vi "TCP Server UnRegister Connection Handler.vi"(8 "error in (no error)":errorcluster, 10 "connection ID":refnum<k5>, 11 "TCP Server RefNum":refnum<class "JKI TCP Server.lvclass">) -> (0 "error out":errorcluster, 1 "Connection Info":T3, 2 "VI References":T2)   [LabVIEW 2020, in "JKI TCP Server.lvclass"]
uses:
  JKI TCP Server.lvclass
  _Data Structures/TCP Server Connection Info Cluster.ctl
  _Data Structures/TCP Server Handler RefNum.ctl
panel:
  # "Copyright © 2004-2008 JKI. All rights reserved.\n\nAuthor: Jim Kring [jim.kring@jameskring.com]\n\nThis library is provided \"AS IS\" ,WITHOUT WARRANTIES OR \nCONDITIONS OF ANY KIND, either express or implied.\n\nJames Kring, Inc. -- http://www.jameskring.com"
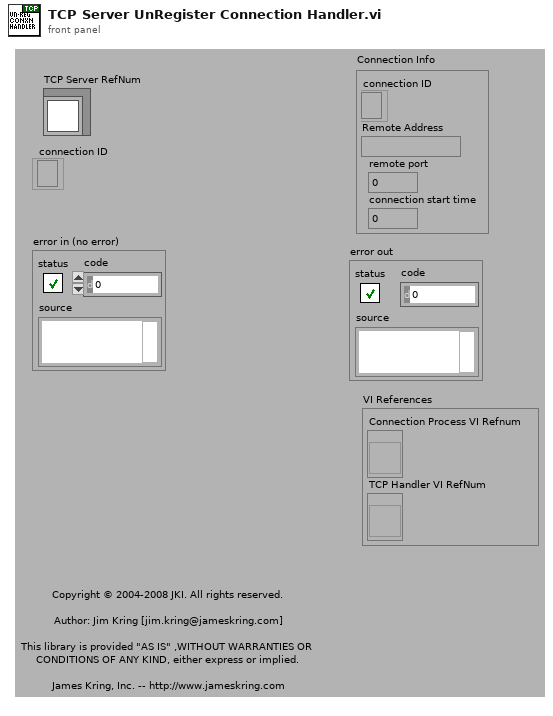
[diagram p1: front panel]
types:
  T1 = typedef "JKI TCP Server.lvclass/TCP Server Handler RefNum.ctl" = refnum<vi>
  T2 = cluster{"Connection Process VI Refnum":refnum<vi>, "TCP Handler VI RefNum":T1}
  T3 = typedef "JKI TCP Server.lvclass/TCP Server Connection Info Cluster.ctl" = cluster{"connection ID":refnum<k5>, "Remote Address":string, "remote port":u16, "connection start time":u32}
  T4 = typedef "JKI TCP Server.lvclass/TCP Server Data.ctl" = cluster{"Listener Info":T5, "Connection Process VI RefNums":refnum<vi>[], "dup connection IDs (for quick search)":refnum<k5>[], "Connections":T3[], "Connection Handler VI Path":path, "Handler Is Reentrant?":bool, "TCP Handler Instance RefNums":T1[], "TCP Handler VI RefNum":T1, "No. Connections":u32, "Max Connections":u32, "server start time":u32, "Additional Data":variant}
  T5 = typedef "JKI TCP Server.lvclass/TCP Server Listener Info Cluster.ctl" = cluster{"listener ID":refnum<k5>, "net address":u32, "port":u16, "Listener Process VI Refnum":refnum<vi>}
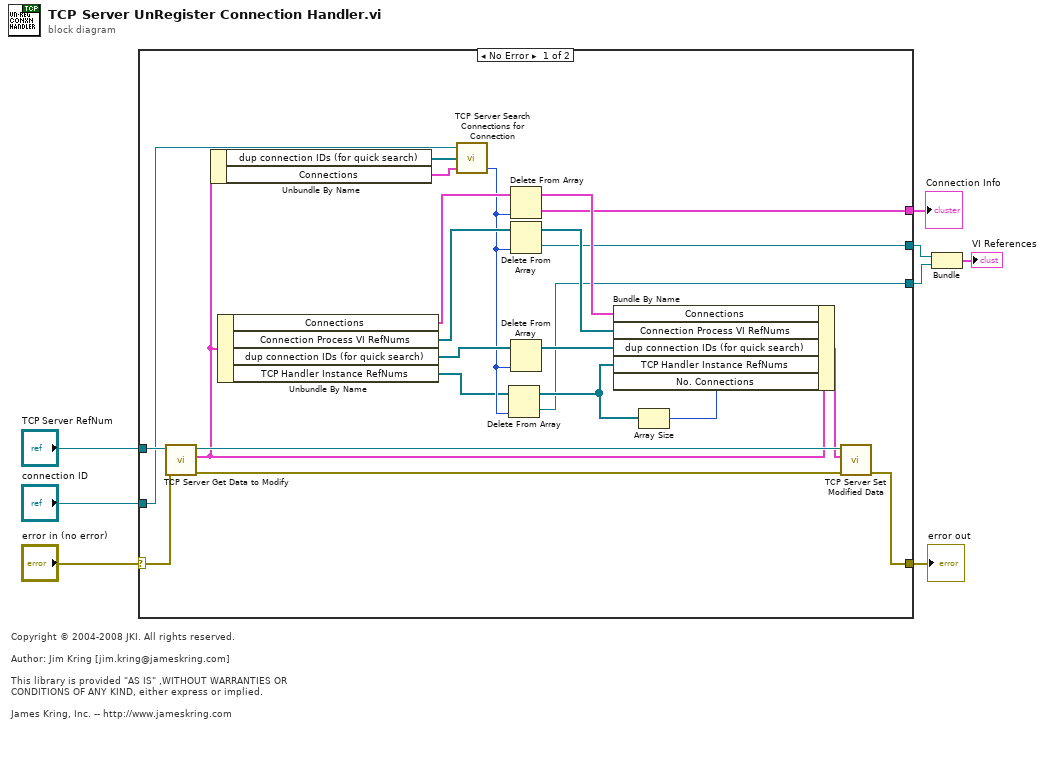
[diagram p0: block diagram]
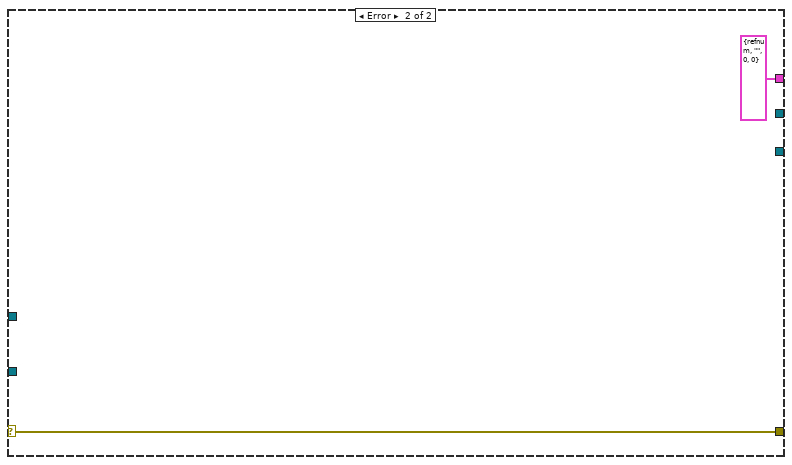
[diagram p2: hidden frame]
diagram:
  # "Copyright © 2004-2008 JKI. All rights reserved.\n\nAuthor: Jim Kring [jim.kring@jameskring.com]\n\nThis library is provided \"AS IS\" ,WITHOUT WARRANTIES OR \nCONDITIONS OF ANY KIND, either express or implied.\n\nJames Kring, Inc. -- http://www.jameskring.com"
  n1 = case shown="No Error" "error in (no error)" {
    tunnel: "TCP Server RefNum" -> [w26 _]
    tunnel: "connection ID" -> [w20 _]
    tunnel: [w28 w33] -> w7
    selector: "error in (no error)" -> [w27 w33]
    tunnel: [w11 T3 {"connection ID"=refnum, "Remote Address"="", "remote port"=0, "connection start time"=0} ("Connection Info")] -> w4
    tunnel: [w10 _] -> w3
    tunnel: [w9 _] -> w2
    frame No Error {
      n2 = call "TCP Server Get Data to Modify.vi"("error in (no error)"=w27, "RefNum"=w26) -> ("error out"=w24:errorcluster, "Data out"=w21:T4, "dup RefNum"=w25:refnum<class "JKI TCP Server.lvclass">)  [unwired: 6 in, 1 out]
      n3 = Unbundle By Name(w21) -> ("dup connection IDs (for quick search)"=w23:refnum<k5>[], "Connections"=w22:T3[])
      n4 = Unbundle By Name(w21) -> ("Connections"=w31:T3[], "Connection Process VI RefNums"=w30:refnum<vi>[], "dup connection IDs (for quick search)"=w19:refnum<k5>[], "TCP Handler Instance RefNums"=w15:T1[])
      n5 = call "TCP Server Search Connections for Connection.vi"("Connections"=w22, "dup connection IDs (for quick search)"=w23, "connection ID"=w20) -> ("index"=w16:i32)  [unwired: 2 out]
      n6 = Delete From Array(array=w15, index=w16) -> (deleted portion=w9:T1, array with subset deleted=w14:T1[])  [unwired: 1 in]
      n7 = Delete From Array(array=w31, index=w16) -> (deleted portion=w11:T3, array with subset deleted=w17:T3[])  [unwired: 1 in]
      n8 = Delete From Array(array=w30, index=w16) -> (deleted portion=w10:refnum<vi>, array with subset deleted=w29:refnum<vi>[])  [unwired: 1 in]
      n9 = Delete From Array(array=w19, index=w16) -> (array with subset deleted=w18:refnum<k5>[])  [unwired: 1 in, 1 out]
      n10 = Array Size(array=w14) -> (size(s)=w13:i32)
      n11 = Bundle By Name(cluster=w21, "Connections"=w17, "Connection Process VI RefNums"=w29, "dup connection IDs (for quick search)"=w18, "TCP Handler Instance RefNums"=w14, "No. Connections"=w13) -> (w12:T4)
      n12 = call "TCP Server Set Modified Data.vi"("error in (no error)"=w24, "Data in"=w12, "RefNum"=w25) -> ("error out"=w28:errorcluster)  [unwired: 7 in, 1 out]
    }
    frame Error {
    }
  }
  "error out" <- w7
  "Connection Info" <- w4
  n13 = Bundle("Connection Process VI Refnum"=w3, "TCP Handler VI RefNum"=w2) -> (→"VI References":T2)  [unwired: 1 in]
